vi "get spectra.vi"() -> ()   [LabVIEW 2013]
uses:
  <vilib>/Utility/file.llb/Write To Spreadsheet File (I64).vi
panel:
  in  "file path":path=path "C:/Users/Ellen/Desktop/Alk Titration trials/junk"
  out "A/D counts":i64[][](array[numeric])
  out "OKH":bool
  in  "’âŽ~":bool=TRUE
  out "XY Graph":cluster{i32[], "Buffer":u16[]}(graph) caption="pixel vs A/D Counts"
  in  "Pixel":u16=1024
  out "OKH":bool
  out "PipeHandle":i32=-1
  out "DeviceHandle":i32=-1
  # "USB_OpenDevice"
  # "USB_OpenPipe"
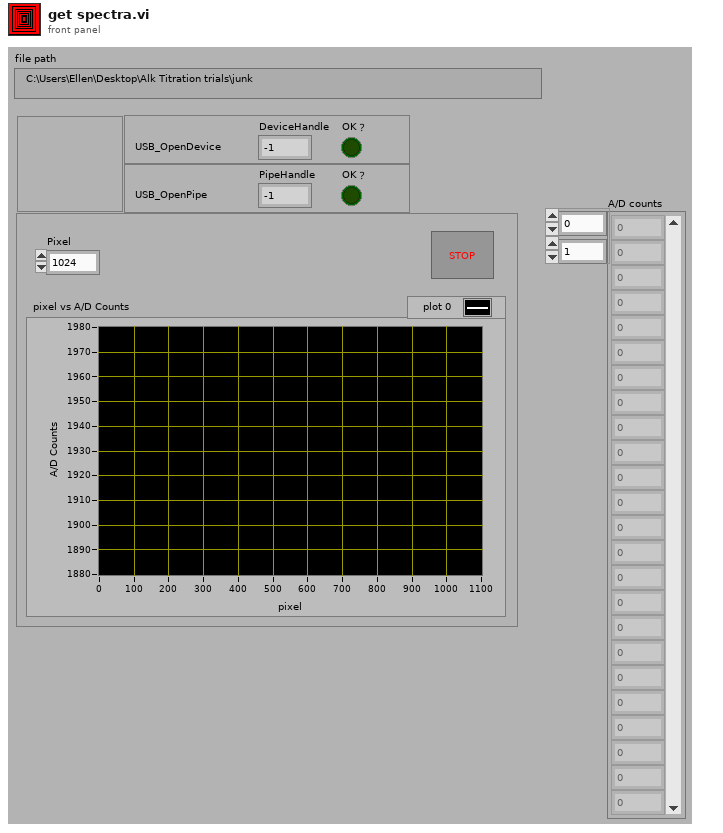
[diagram p1: front panel]
types:
  T1 = typedef "specu1a 1.0.0 Product Information.ctl" = cluster{"UnitID":string, "Sensor Name":string, "Serial Number":string, "Reserved":string, "Wave Upper":u16, "Wave Lower":u16}
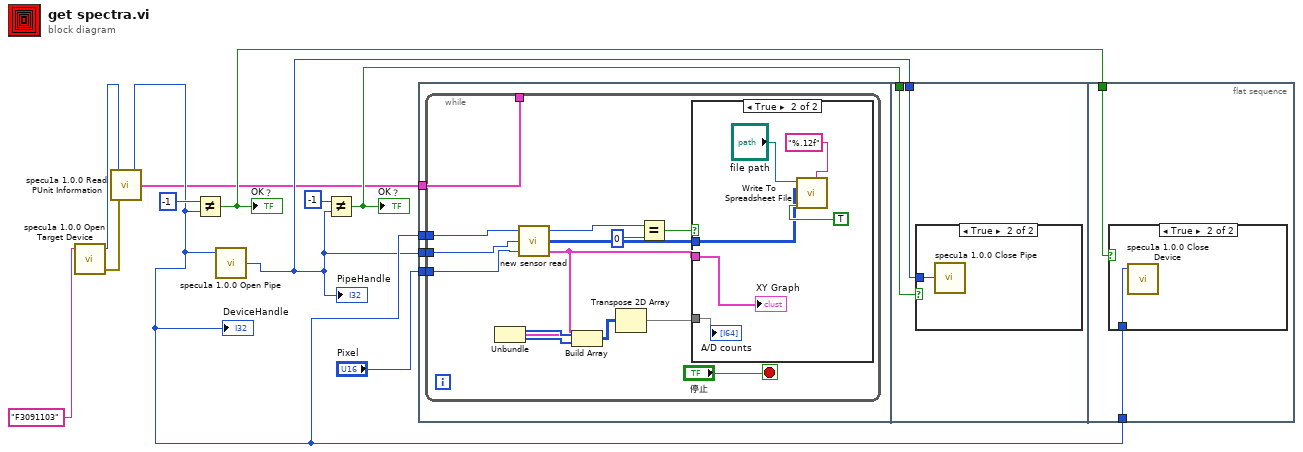
[diagram p0: block diagram]
diagram:
  n1 = call <instrlib>:"specu1a 1.0.0 Open Target Device.vi"("Unit ID"="F3091103") -> ("error out"=w4:errorcluster, "Device Handle"=w5:i32)  [unwired: 2 in, 1 out]
  n2 = call <instrlib>:"specu1a 1.0.0 Read PUnit Information.vi"("error in (no error)"=w4, "Device Handle"=w5) -> ("Unit Information out"=w1:T1, "Device Handle out"=w3:i32)  [unwired: 1 in, 1 out]
  "DeviceHandle" <- w3
  n3 = Not Equal?(x=-1, y=w3) -> (x != y?=w9:bool)
  "OKH" <- w9
  n4 = call <instrlib>:"specu1a 1.0.0 Open Pipe.vi"("Device Handle"=w3) -> ("Pipe Handle"=w2:i32)  [unwired: 2 in, 2 out]
  "PipeHandle" <- w2
  n5 = Not Equal?(x=-1, y=w2) -> (x != y?=w8:bool)
  "OKH" <- w8
  n6 = flat-sequence {
    tunnel: w3 -> [w15]
    tunnel: w2 -> [w14]
    tunnel: "Pixel" -> [w13]
    tunnel: w1 -> [w12]
    tunnel: w8 -> [w36]
    tunnel: w2 -> [w35]
    tunnel: w3 -> [w39]
    tunnel: w9 -> [w38]
    frame #0 {
      n7 = while {
        tunnel: w15 -> [w24]
        tunnel: w14 -> [w23]
        tunnel: w13 -> [w22]
        tunnel: w12 -> [_]
        stop <- "’âŽ~" stop-if-true
        n8 = call <instrlib>:"new sensor read.vi"("Device Handle 2"=w24, "Pipe handle"=w23, "PixelSize"=w22) -> ("return type"=w25:u16, "appended array"=w16:u16[][], "XY Graph"=w18:cluster{i32[], "Buffer":u16[]})  [unwired: 4 in]
        n9 = Unbundle(w18) -> (w20:i32[], "Buffer"=w19:u16[])
        n10 = Build Array(w20, w19) -> (w21:i32[][])
        n11 = Transpose 2D Array(2D array=w21) -> (transposed array=w17:i32[][])
        n12 = Equal?(x=w25, y=0) -> (x = y?=w28:bool)
        n13 = case shown="True" w28 {
          tunnel: w18 -> [_ w34]
          tunnel: w17 -> [_ w33]
          tunnel: w16 -> [_ w29]
          frame False {
          }
          frame True {
            n14 = call-poly <vilib>:"Write To Spreadsheet File.vi"("format (%d)"="%.12f" ("format (%.3f)"), "append to file? (new file:F)"=TRUE, "2D data"=w29, "file path (dialog if empty)"="file path") -> ()  [unwired: 4 in, 1 out]
            "XY Graph" <- w34
            "A/D counts" <- w33
          }
        }
      }
    }
    frame #1 {
      n15 = case shown="True" w36 {
        tunnel: w35 -> [_ w37]
        frame False {
        }
        frame True {
          n16 = call <instrlib>:"specu1a 1.0.0 Close Pipe.vi"("Pipe Handle"=w37) -> ()  [unwired: 3 in, 2 out]
        }
      }
    }
    frame #2 {
      n17 = case shown="True" w38 {
        tunnel: w39 -> [_ w40]
        frame False {
        }
        frame True {
          n18 = call <instrlib>:"specu1a 1.0.0 Close Device.vi"("Device Handle"=w40) -> ()  [unwired: 4 in, 1 out]
        }
      }
    }
  }
